vi "find and draw circles.vi"(0 "Image Src":T1, 1 "module path":path, 2 "function name":string="get_circels", 3 "initialized array":dbl[][](array[numeric]), 4 "Image Dst":T1, 5 "error in (no error)":errorcluster, 6 "session in":refnum<k35>, 7 "Run/Stop":bool, 8 "grading Thr":dbl[](array[numeric])) -> (14 "session out":refnum<k35>, 15 "circle info":dbl[][](array[numeric]), 16 "Image Out":T1, 18 "error out":errorcluster, 19 "pellet detected?":bool)   [LabVIEW 2019]
uses:
  <vilib>/vision/Image Controls.llb/IMAQ Image.ctl
  <vilib>/Utility/error.llb/DialogType.ctl
  detectedPellet.lvlib
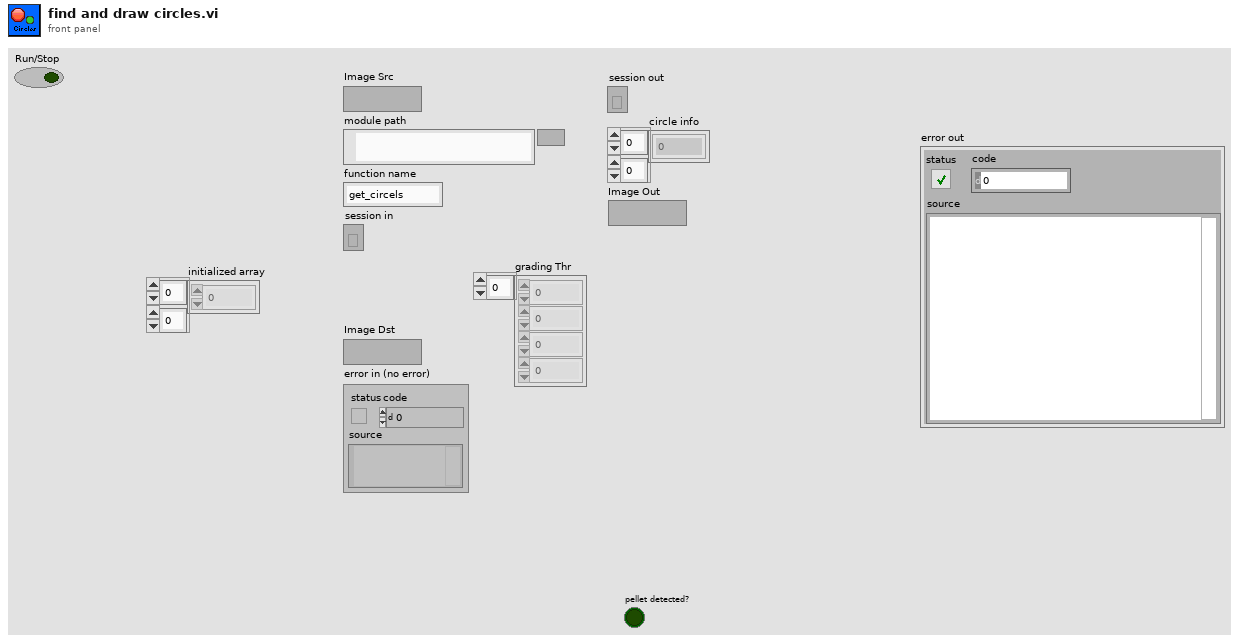
[diagram p1: front panel]
types:
  T1 = typedef "IMAQ Image.ctl" = refnum<image>
  T2 = typedef "DialogType.ctl" = u16
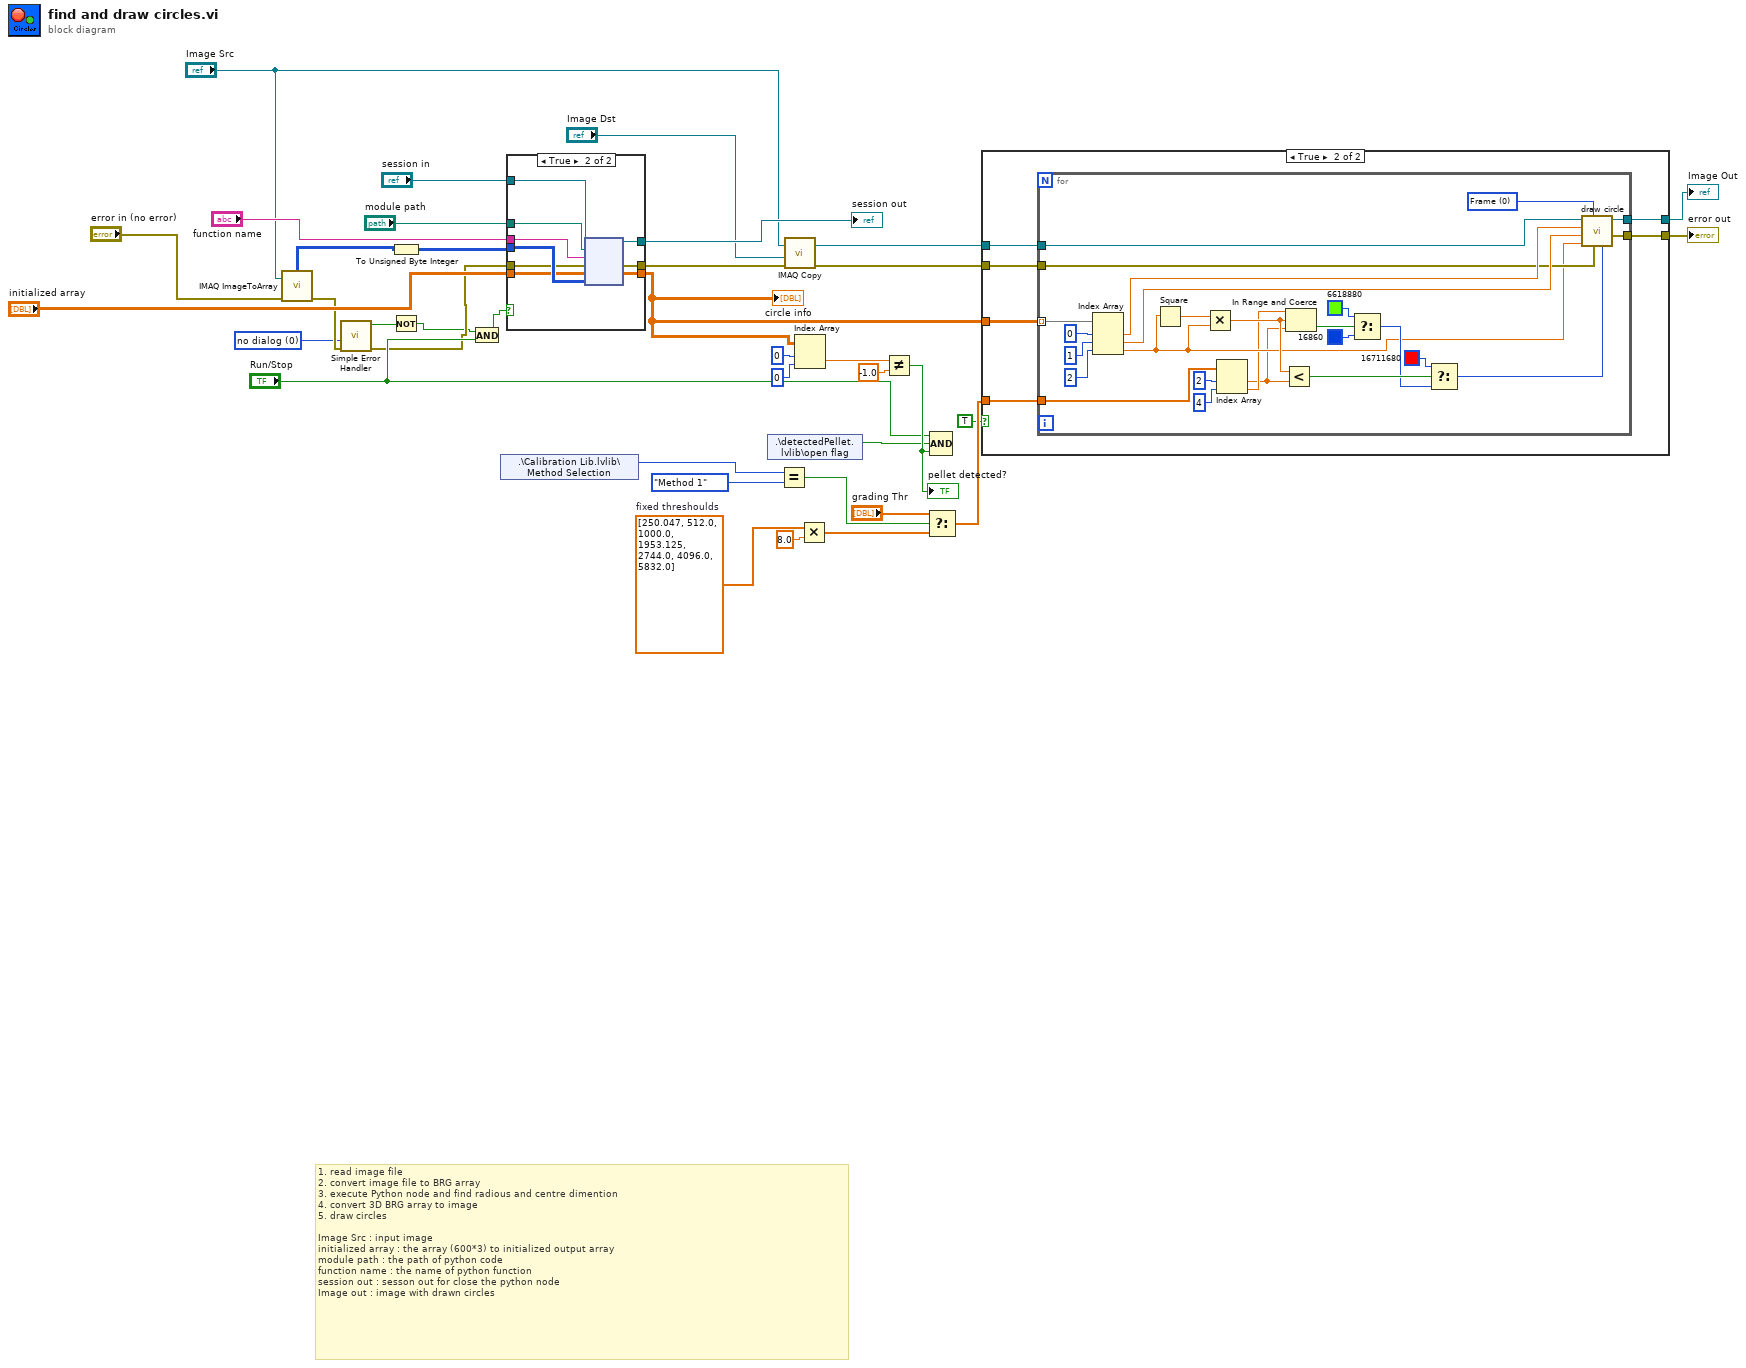
[diagram p0: block diagram]
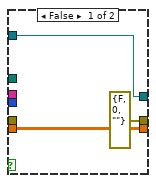
[diagram p2: hidden frame]
diagram:
  w5 = T2 0 items=["no dialog", "OK message", "continue or stop message", "OK message + warnings", "continue/stop + warnings"] ("type of dialog (OK msg:1)")
  w20 = dbl[] [250.047, 512.0, 1000.0, 1953.125, 2744.0, 4096.0, 5832.0]  # fixed threshoulds
  # "1. read image file\n2. convert image file to BRG array\n3. execute Python node and find radious and centre dimention\n4. convert 3D BRG array to image\n5. draw circles\n\nImage Src : input image\ninitialized array : the array (600*3) to initialized output array \nmodule path : the path of python code\nfunction name : the name of python function \nsession out : sesson out for close the python node\nImage out : image with drawn circles"
  n1 = call "IMAQ ImageToArray"("error in (no error)"="error in (no error)", "Image"="Image Src") -> ("error out"=w9:errorcluster, "Image Pixels (U8)"=w2:u8[][])  [unwired: 2 in, 3 out]
  n2 = call <vilib>:"Simple Error Handler.vi"("type of dialog (OK msg:1)"=w5, "error in (no error)"=w9) -> ("error?"=w4:bool, "error out"=w6:errorcluster)  [unwired: 3 in, 3 out]
  n3 = To Unsigned Byte Integer(number=w2) -> (unsigned 8bit integer=w1:u8[][])
  n4 = Not(x=w4) -> (.not. x?=w3:bool)
  n5 = And(x=w3, y="Run/Stop") -> (x .and. y?=w7:bool)
  n6 = shared-variable ".\\Calibration Lib.lvlib\\Method Selection"() -> (w21:enum32{"Method 1", "Method 2"})  [unwired: 1 in, 1 out]
  n7 = case shown="True" w7 {
    tunnel: "module path" -> [_ w50]
    tunnel: "function name" -> [_ w49]
    tunnel: w1 -> [_ w48]
    tunnel: [w41 w47] -> w35
    tunnel: "initialized array" -> [w40 w46]
    tunnel: [errorcluster {"status"=FALSE, "code"=0, "source"=""} ("function name out") w45] -> w32
    tunnel: "session in" -> [w41 w44]
    tunnel: [w40 w43] -> w12
    tunnel: w6 -> [_ w42]
    frame False {
    }
    frame True {
      n8 = node(w44, w50, w49, w42, w46, w48) -> (w47:refnum<k35>, w45:errorcluster, w43:dbl[][])  [unwired: 1 in, 2 out]
    }
  }
  "session out" <- w35
  "circle info" <- w12
  n9 = shared-variable ".\\detectedPellet.lvlib\\open flag"() -> (w15:bool)  [unwired: 1 in, 1 out]
  n10 = Equal?(x=w21, y=enum32{"Method 1", "Method 2"}."Method 1" ("Method Selection")) -> (x = y?=w22:bool)
  n11 = call "IMAQ Copy"("error in (no error)"=w32, "Image Dst"="Image Dst", "Image Src"="Image Src") -> ("error out"=w36:errorcluster, "Image Dst Out"=w30:T1)  [unwired: 3 in]
  n12 = Index Array(array=w12, index (row)=0, index (col)=0 ("disabled index (col)")) -> (element=w27:dbl)
  n13 = Multiply(x=w20, y=8.0) -> (x*y=w19:dbl[])
  n14 = Not Equal?(x=w27, y=-1.0) -> (x != y?=w25:bool)
  "pellet detected?" <- w25
  n15 = Select(t="grading Thr", s=w22, f=w19) -> (s? t:f=w16:dbl[])
  n16 = Compound Arithmetic op=AND("Run/Stop", w15, w25) -> ()  [unwired: 1 out]
  n17 = case shown="True" TRUE {
    tunnel: w36 -> [w51 w58]
    tunnel: w12 -> [_ w57]
    tunnel: [w51 w56] -> w34
    tunnel: w30 -> [w52 w55]
    tunnel: [w52 w54] -> w24
    tunnel: w16 -> [_ w53]
    frame False {
    }
    frame True {
      n18 = for {
        tunnel: w55 -> [w84]
        tunnel: w57 -> [w83] mode=indexing
        tunnel: w58 -> [w76]
        tunnel: [w75] -> w56
        tunnel: [w74] -> w54
        tunnel: w53 -> [w61]
        w77 = u32 0 items=["Frame", "Fill"] ("Drawing Mode (Frame)")
        n19 = Index Array(array=w83, index #1=0 ("index"), index #2=1 ("index"), index #3=2 ("index")) -> (element #1=w79:dbl, element #2=w78:dbl, element #3=w62:dbl)
        n20 = Square(x=w62) -> (x^2=w73:dbl)
        n21 = Multiply(x=w73, y=w62) -> (x*y=w69:dbl)
        n22 = Index Array(array=w61, index #1=2 ("index"), index #2=4 ("index")) -> (element #1=w59:dbl, element #2=w60:dbl)
        n23 = Less?(x=w69, y=w59) -> (x < y?=w71:bool)
        n24 = In Range and Coerce(upper limit=w60, x=w69, lower limit=w59) -> (In Range?=w67:bool)  [unwired: 1 out]
        n25 = Select(t=u32 6618880 ("Color 2"), s=w67, f=u32 16860 ("Color 2")) -> (s? t:f=w64:u32)
        n26 = Select(t=u32 16711680 ("Color"), s=w71, f=w64) -> (s? t:f=w63:u32)
        n27 = call "draw circle.vi"("Color"=w63, "error in (no error)"=w76, "Drawing Mode (Frame)"=w77, "box size"=w62, "Y"=w78, "X"=w79, "Image In"=w84) -> ("error out"=w75:errorcluster, "Image Out"=w74:T1)  [unwired: 3 in]
      }
    }
  }
  "Image Out" <- w24
  "error out" <- w34
